vi "DynamicScanLinitParser.vi"() -> ()   [LabVIEW 2018]
panel:
  out "element 6":string
  out "freq_lsl":string
  out "freq_hsl":string
  out "pow_lsl":string
  out "pow_hsl":string
  out "element":string
  out "array":string[](array[string])
  out "text":string
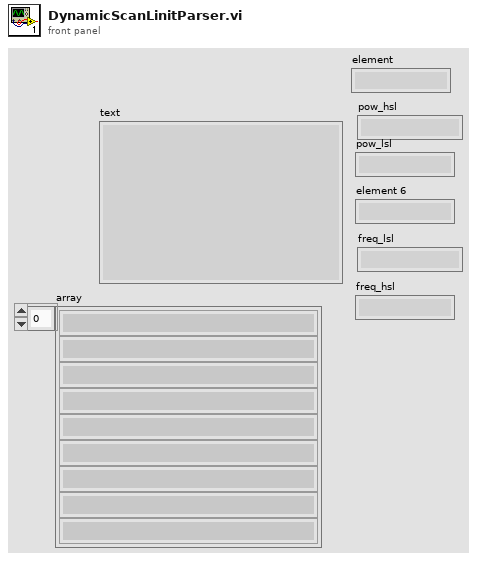
[diagram p1: front panel]
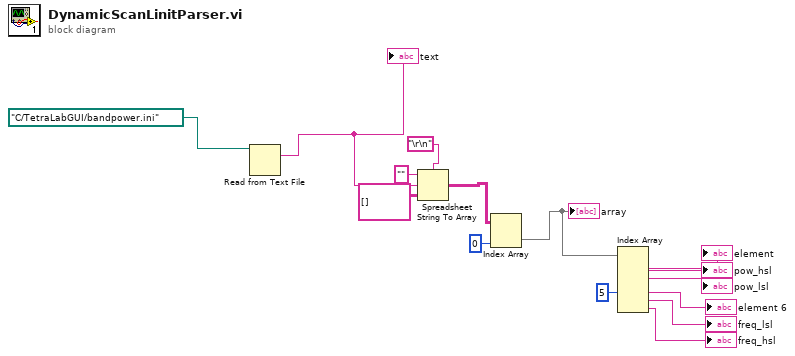
[diagram p0: block diagram]
diagram:
  n1 = Read from Text File(file (use dialog)=path "C:/TetraLabGUI/bandpower.ini") -> (text=w9:string)  [unwired: 3 in, 3 out]
  "text" <- w9
  n2 = Spreadsheet String To Array(delimiter (Tab)="\r\n", format string="", spreadsheet string=w9, array type (2D Dbl)=string[][] []) -> (array=w11:string[][])
  n3 = Index Array(array=w11, index (col)=0 ("disabled index (col)")) -> (element=w8:string[])  [unwired: 1 in]
  "array" <- w8
  n4 = Index Array(array=w8, index #4=5 ("index")) -> (element #1=→"element":string, element #2=→"pow_hsl":string, element #3=→"pow_lsl":string, element #4=→"element 6":string, element #5=→"freq_lsl":string, element #6=→"freq_hsl":string)  [unwired: 5 in]
